vi "FPGA Phasor Measurement for M Class (60 Hz).vi"(0 "signal in":fxp<+/-,24,1>, 1 "number of channels":T3=1 items=["1"=1, "2"=2, "3"=3, "4"=4, "5"=5, "6"=6, "7"=7, "8"=8, "9"=9, "10"=10, "11"=11, "12"=12, "13"=13, "14"=14, "15"=15, "16"=16], 2 "memory information":T1, 5 "timestamp [s]":fxp<+,64,32> format="%#_42g", 7 "reference channel index (0)":u8, 9 "input valid? (T)":bool=TRUE, 12 "ready for output? (T)":bool=TRUE) -> (4 "output data":T2 {"timestamp [s]" format="%#.6g"; "phase [pi]" format="%#.6g"}, 10 "output valid?":bool, 14 "ready for input?":bool, 15 "error":i32)   [LabVIEW 2014, in "NI_EP_PMU_FPGA.lvlib"]
doc: "Calculates the instantaneous magnitude, phase, and frequency values of the fundamental frequency component as defined in the M class of performance in IEEE Std C37.118.1-2011. This VI resamples even-time-spaced voltage and current signals into even-angle-spaced signals. The input signals must have a sample rate of 50 kHz. The output rate is 24 samples per cycle. You must manually select the polymorphic instance to use."
uses:
  <vilib>/addons/Electrical Power/PMU/NI_EP_PMU_FPGA.lvlib
  <vilib>/addons/Electrical Power/PQ/Resampling/FPGA/subVIs/fpga_NofCH.ctl
  <vilib>/addons/Electrical Power/PQ/Resampling/NI_EP_Resample_FPGA.lvlib
  <vilib>/addons/Electrical Power/PMU/FPGA/subVIs/fpga_OutputDataType.ctl
  <vilib>/addons/Electrical Power/PMU/FPGA/subVIs/fpga_Memory Information (M Class_60Hz).ctl
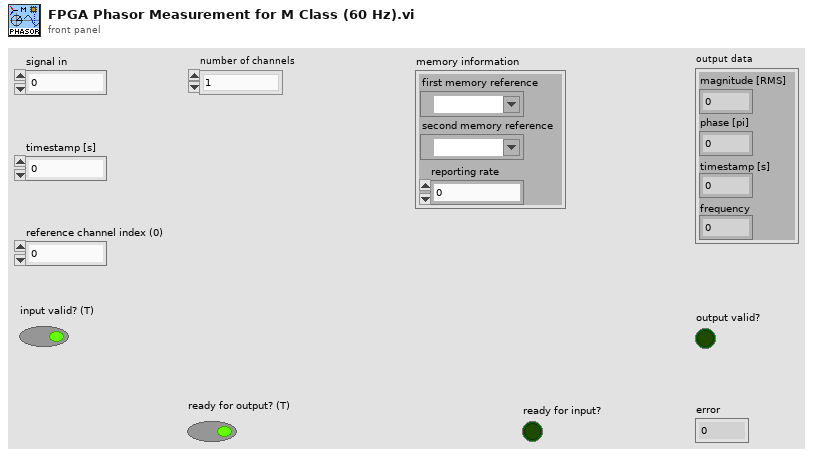
[diagram p1: front panel]
types:
  T1 = typedef "NI_EP_PMU_FPGA.lvlib/fpga_Memory Information (M Class_60Hz).ctl" = cluster{"first memory reference":refnum<k21>, "second memory reference":refnum<k21>, "reporting rate":i16}
  T2 = typedef "NI_EP_PMU_FPGA.lvlib/fpga_OutputDataType.ctl" = cluster{"magnitude [RMS]":fxp<+,32,6>, "phase [pi]":fxp<+/-,32,2>, "timestamp [s]":fxp<+,64,32>, "frequency":fxp<+,32,8>}
  T3 = typedef "NI_EP_Resample_FPGA.lvlib/fpga_NofCH.ctl" = u8
  T4 = typedef "NI_EP_Resample_FPGA.lvlib/fpga_Resampled.ctl" = cluster{"signal":fxp<+/-,32,3>, "timestamp [s]":fxp<+,64,32>, "frequency":fxp<+,32,8>}
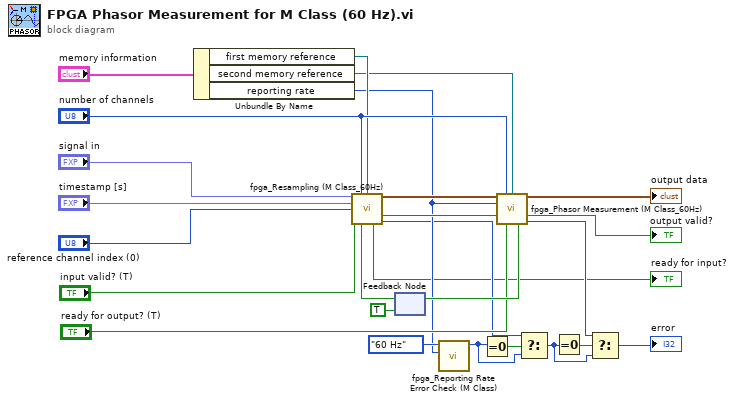
[diagram p0: block diagram]
diagram:
  n1 = Unbundle By Name("memory information") -> ("first memory reference"=w15:refnum<k21>, "second memory reference"=w14:refnum<k21>, "reporting rate"=w9:i16)
  n2 = feedback #1(TRUE ("ready for input")) -> (w18:bool)
  n3 = call <vilib>:"fpga_Resampling (M Class_60Hz).vi"("signal in"="signal in", "number of channels"="number of channels", "Memory In"=w15, "timestamp [s]"="timestamp [s]", "reference channel index"="reference channel index (0)", "input data valid? (T)"="input valid? (T)", "ready for output? (T)"=w18) -> ("resampled data"=w23:T4, "output valid"=w22:bool, "ready for input"=→"ready for input?":bool, "error"=w6:i32)  [unwired: 5 in]
  n4 = call <vilib>:"fpga_Reporting Rate Error Check (M Class).vi"("reporting rate"=w9, "nominal frequency"=enum16{"50 Hz", "60 Hz"}."60 Hz") -> ("error"=w7:i32)  [unwired: 9 in]
  n5 = Equal To 0?(x=w7) -> (x = 0?=w8:bool)
  n6 = call <vilib>:"fpga_Phasor Measurement (M Class_60Hz).vi"("resampled data"=w23, "number of channels"="number of channels", "Memory In"=w14, "reporting rate"=w9, "input valid? (T)"=w22, "ready for output? (T)"="ready for output? (T)") -> ("output data"=→"output data":T2, "output valid"=→"output valid?":bool, "ready for input"=w20:bool, "error"=w3:i32)  [unwired: 6 in]
  n7 = feedback-in #1(w20) -> ()
  n8 = Select(t=w6, s=w8, f=w7) -> (s? t:f=w4:i32)
  n9 = Equal To 0?(x=w4) -> (x = 0?=w5:bool)
  n10 = Select(t=w3, s=w5, f=w4) -> (s? t:f=→"error":i32)
